vi "button(sub vi).vi"(11 "1":bool[](array[boolean])) -> (0 "2":dbl, 1 "1":dbl, 2 "2":bool, 3 "1":bool)   [LabVIEW 2017]
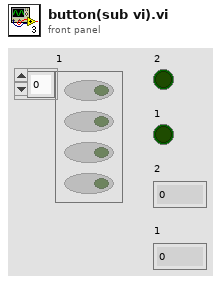
[diagram p1: front panel]
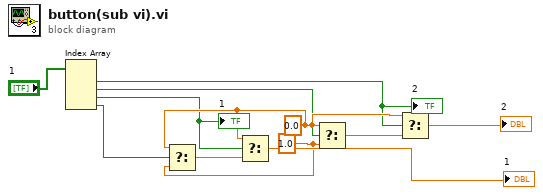
[diagram p0: block diagram]
diagram:
  w7 = 1.0 ("f")
  w11 = 0.0 ("t")
  n1 = Index Array(array="1") -> (element #1=w6:bool, element #2=w5:bool, element #3=w4:bool, element #4=w3:bool)  [unwired: 4 in]
  "2" <- w6
  "1" <- w4
  n2 = Select(t=w11, s=w3, f=w7) -> (s? t:f=w1:dbl)
  n3 = Select(t=w11, s=w4, f=w1) -> (s? t:f=→"1":dbl)
  n4 = Select(t=w11, s=w5, f=w7) -> (s? t:f=w2:dbl)
  n5 = Select(t=w11, s=w6, f=w2) -> (s? t:f=→"2":dbl)
